vi "NF87XX.lock.vi"(0 "i ref in":refnum<vi>, 5 "error in (no error)":errorcluster) -> (14 "i ref out":refnum<vi>, 19 "error out":errorcluster)   [LabVIEW 2014, in "NF87XX.lvlib"]
doc: "This command issued from any connected input device locks out all other connected devices.\n\nauthor: Stefan Götte\ndata: 30-AUG-2006\n\n\nLicense Agreement for this software:\n\nCopyright (C)\nGesellschaft für Schwerionenforschung, GSI\nPlanckstr. 1\n64291 Darmstadt\nGermany\n\nContact: D.Beck@gsi.de \n\nThis program is free software; you can redistribute it and/or modify it under the terms of the GNU General Public License as published by the Free Software Foundation; either version 2 of the license, or (at your option) any later version.\n\nThis program is distributed in the hope that it will be useful, but WITHOUT ANY WARRANTY; without even the implied warranty of MERCHANTABILITY or FITNESS FOR A PARTICULAR PURPOSE. See the GNU General License for more details (http://www.gnu.org).\n\nGesellschaft für Schwerionenforschung, GSI\nPlanckstr. 1, 64291 Darmstadt, Germany\nFor all questions and ideas contact: M.Richter@gsi.de, H.Brand@gsi.de or D.Beck@gsi.de.\nLast update: 17-JUN-2004"
uses:
  NF87XX.lvlib
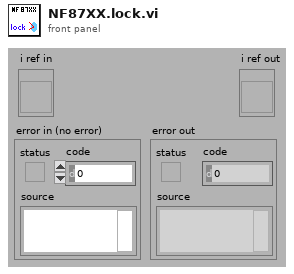
[diagram p1: front panel]
types:
  T1 = enum16{"User....", "DEF", "DIAG", "INI", "LOCK", "UNLOCK", "MAP", "SAV", "VER", "ACC", "CHL", "FOR", "GO", "HAL", "MOF", "MON", "MPV", "POS", "REL", "REV", "STA", "STO", "TYP", "VEL", "ABS", "SER", "NOS", "DRT", "FLI", "RLI", "FIN", "RIN", "AIN", "IN", "JOF", "JON", "OUT", "RES FINE", "RES COARSE", "02 (HEX)", "PWM", "CNT", "TMR", "HOSTNAME", "IPADDR", "IPMODE", "NETMASK", "GATEWAY", "DNSSRVR", "PASSWD", "ECHO", "MACADDR"}
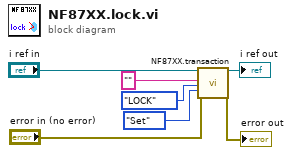
[diagram p0: block diagram]
diagram:
  n1 = call "NF87XX.transaction.vi"("i ref in"="i ref in", "User Cmd/Numeric Argu"="", "MCL Cmd"=T1."LOCK", "Query/Set"=enum16{"Query", "Set"}."Set", "error in (no error)"="error in (no error)") -> ("i ref out"=→"i ref out":refnum<vi>, "error out"=→"error out":errorcluster)  [unwired: 12 in, 1 out]
